vi "Subvi iterator.vi"(9 "Set increase":bool, 10 "Iterator in":i32, 11 "Nmax":i32) -> (0 "Stop":bool, 2 "Iterator out":i32)   [LabVIEW 2017]
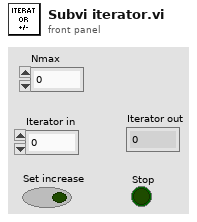
[diagram p1: front panel]
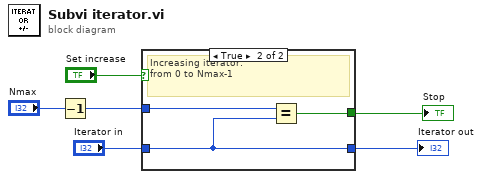
[diagram p0: block diagram]
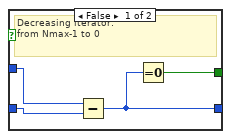
[diagram p2: hidden frame]
diagram:
  n1 = Decrement(x="Nmax") -> (x-1=w1:i32)
  n2 = case shown="True" "Set increase" {
    tunnel: [w8 w13] -> w5
    tunnel: "Iterator in" -> [w9 w12]
    tunnel: [w7 w12] -> w3
    tunnel: w1 -> [w10 w11]
    frame False {
      # "Decreasing iterator:\nfrom Nmax-1 to 0"
      n3 = Subtract(x=w10, y=w9) -> (x-y=w7:i32)
      n4 = Equal To 0?(x=w7) -> (x = 0?=w8:bool)
    }
    frame True {
      # "Increasing iterator:\nfrom 0 to Nmax-1"
      n5 = Equal?(x=w11, y=w12) -> (x = y?=w13:bool)
    }
  }
  "Stop" <- w5
  "Iterator out" <- w3
